vi "z1.vi"() -> ()   [LabVIEW 2013]
uses:
  kernel32.dll
panel:
  out "return type":i32
  out "lpnSize":u32
  out "lpBuffer":string
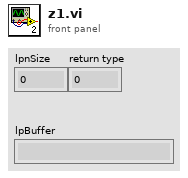
[diagram p1: front panel]
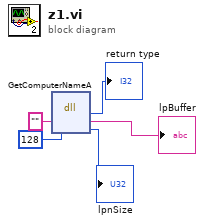
[diagram p0: block diagram]
diagram:
  n1 = dll-call lib="kernel32.dll" fn="GetComputerNameA"("lpBuffer"="", "lpnSize"=u32 128) -> ("return type"=→"return type":i32, "lpBuffer"=→"lpBuffer":string, "lpnSize"=→"lpnSize":u32)  [unwired: 3 in, 2 out]
